vi "Destroy Publish Data Events.vi"(8 "error in (no error)":errorcluster, 11 "UserEvents in":refnum<class "User Events.lvclass">) -> (0 "error out":errorcluster, 3 "UserEvents out":refnum<class "User Events.lvclass">)   [LabVIEW 2016, in "User Events.lvclass"]
uses:
  User Events.lvclass
  User Events.lvclass/User Events.ctl
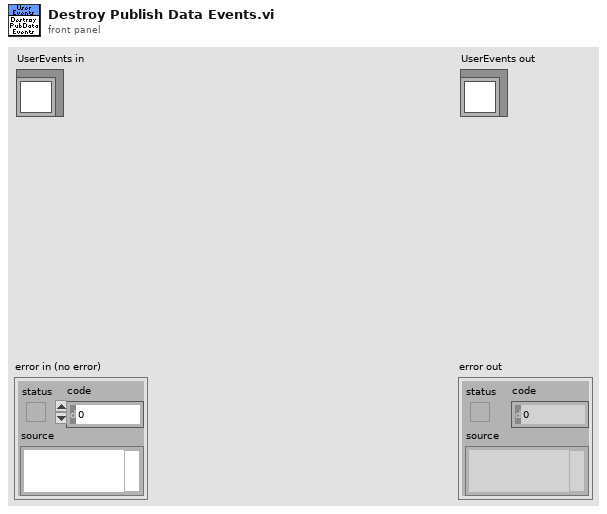
[diagram p1: front panel]
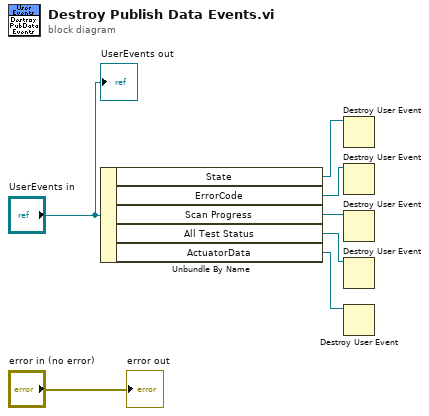
[diagram p0: block diagram]
diagram:
  n1 = Unbundle By Name("UserEvents in") -> ("State"=w6:refnum<user-event>, "ErrorCode"=w5:refnum<user-event>, "Scan Progress"=w4:refnum<user-event>, "All Test Status"=w2:refnum<user-event>, "ActuatorData"=w1:refnum<user-event>)
  n2 = Destroy User Event(user event=w6) -> ()  [unwired: 1 in, 1 out]
  n3 = Destroy User Event(user event=w5) -> ()  [unwired: 1 in, 1 out]
  n4 = Destroy User Event(user event=w4) -> ()  [unwired: 1 in, 1 out]
  n5 = Destroy User Event(user event=w2) -> ()  [unwired: 1 in, 1 out]
  n6 = Destroy User Event(user event=w1) -> ()  [unwired: 1 in, 1 out]
  "error out" <- "error in (no error)"
  "UserEvents out" <- "UserEvents in"
